vi "UIRef.vi"(8 "error in":errorcluster, 11 "tag bus configurable plugin editor node in":refnum<class "tag bus configurable plugin editor node.lvclass">) -> (0 "error out":errorcluster, 2 "VI refnum":refnum<vi>, 3 "tag bus configurable plugin editor node out":refnum<class "tag bus configurable plugin editor node.lvclass">)   [LabVIEW 2014, in "tag bus configurable plugin editor node.lvclass"]
uses:
  tag bus configurable plugin editor node.lvclass
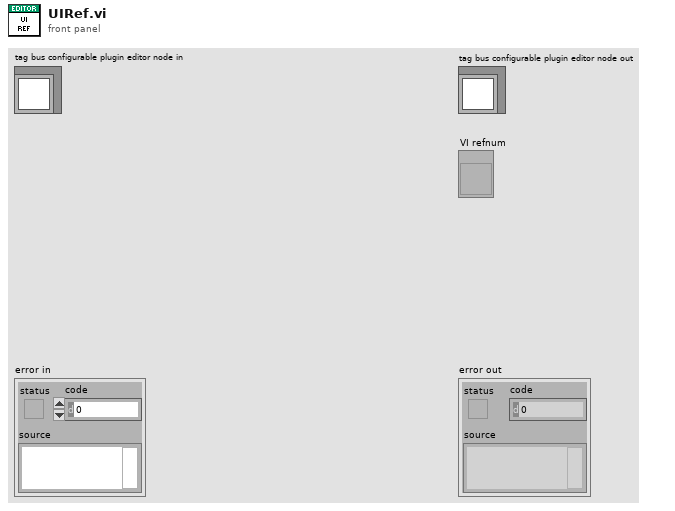
[diagram p1: front panel]
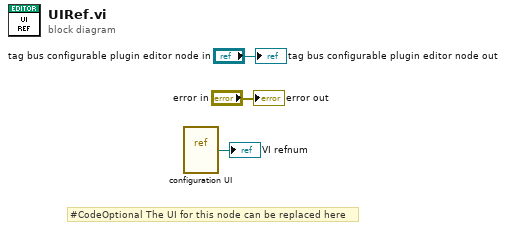
[diagram p0: block diagram]
diagram:
  # "#CodeOptional The UI for this node can be replaced here"
  n1 = vi-ref "configuration UI.vi"() -> (→"VI refnum":refnum<vi>)
  "error out" <- "error in"
  "tag bus configurable plugin editor node out" <- "tag bus configurable plugin editor node in"
